vi "Convert SN data to SN bytes.vi"(11 "SN":u32) -> (3 "Data bytes":u8[](array[numeric]) format="%.0x")   [LabVIEW 2025]
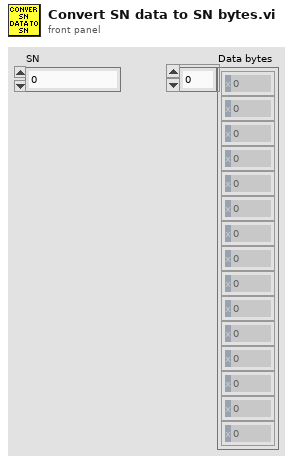
[diagram p1: front panel]
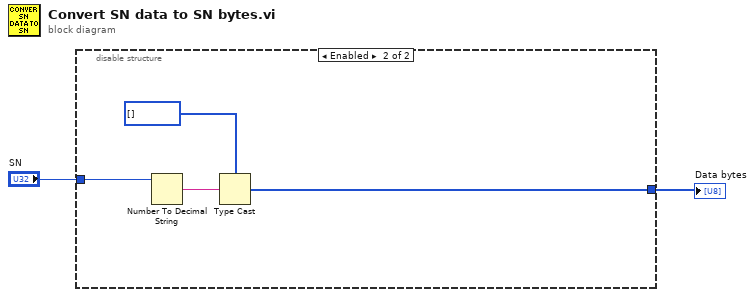
[diagram p0: block diagram]
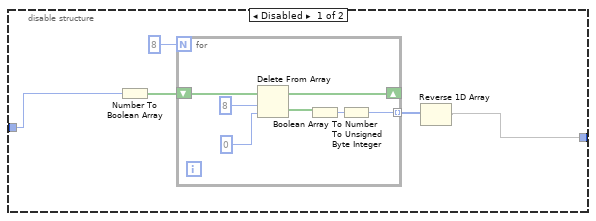
[diagram p2: hidden frame]
diagram:
  n1 = disable-structure shown="Enabled" {
    disable-tunnel: "SN" -> [w4 w16]
    disable-tunnel: [w3 w15] -> w1
    frame Disabled {
      n2 = Number To Boolean Array(number=w4) -> (Boolean array=w7:bool[])
      n3 = for {
        N: 8 -> [_]
        shift-right: [w14] -> _
        shift-left: w7 -> [w13]
        tunnel: [w8] -> w5 mode=indexing
        n4 = Delete From Array(array=w13, length=8, index=0) -> (deleted portion=w10:bool[], array with subset deleted=w14:bool[])
        n5 = Boolean Array To Number(Boolean array=w10) -> (number=w9:u32)
        n6 = To Unsigned Byte Integer(number=w9) -> (unsigned 8bit integer=w8:u8)
      }
      n7 = Reverse 1D Array(array=w5) -> (reversed array=w3:u8[])
    }
    frame Enabled {
      n8 = Number To Decimal String(number=w16) -> (decimal integer string=w17:string)  [unwired: 1 in]
      n9 = Type Cast(type=u8[] [] ("DATA[5]"), x=w17) -> (*(type *) &x=w15:u8[])
    }
  }
  "Data bytes" <- w1
